vi "WPI_RobotDriveOpen4Wheel.vi"   [LabVIEW 2017]
doc: "Opens a reference to the motors you indicate and specifies the responsiveness of the joystick to the motors. You must open a reference before using any other VIs on this palette.\n\nThis software is licensed. Open the labview\\readme\\WPI Robotics Library Open Source License.txt file for more information."
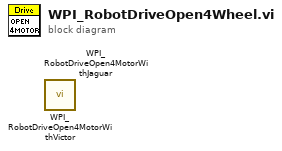
[diagram p0: block diagram]
diagram:
  n1 = call <vilib>:"WPI_RobotDriveOpen4MotorWithVictor.vi"() -> ()  [unwired: 14 in, 2 out]
  n2 = call <vilib>:"WPI_RobotDriveOpen4MotorWithJaguar.vi"() -> ()  [unwired: 14 in, 2 out]
